vi "Encoder Control Logic.vi"(8 "Prev Phase B (State Bit 1)":bool, 9 "Prev Phase A (State Bit 0)":bool, 10 "Phase B":bool, 11 "Phase A":bool) -> (1 "Count?":bool, 2 "Backward?":bool, 3 "Error Occurred?":bool, 4 "deltaT":i32)   [LabVIEW 2017]
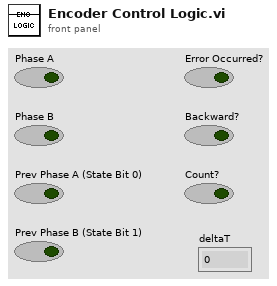
[diagram p1: front panel]
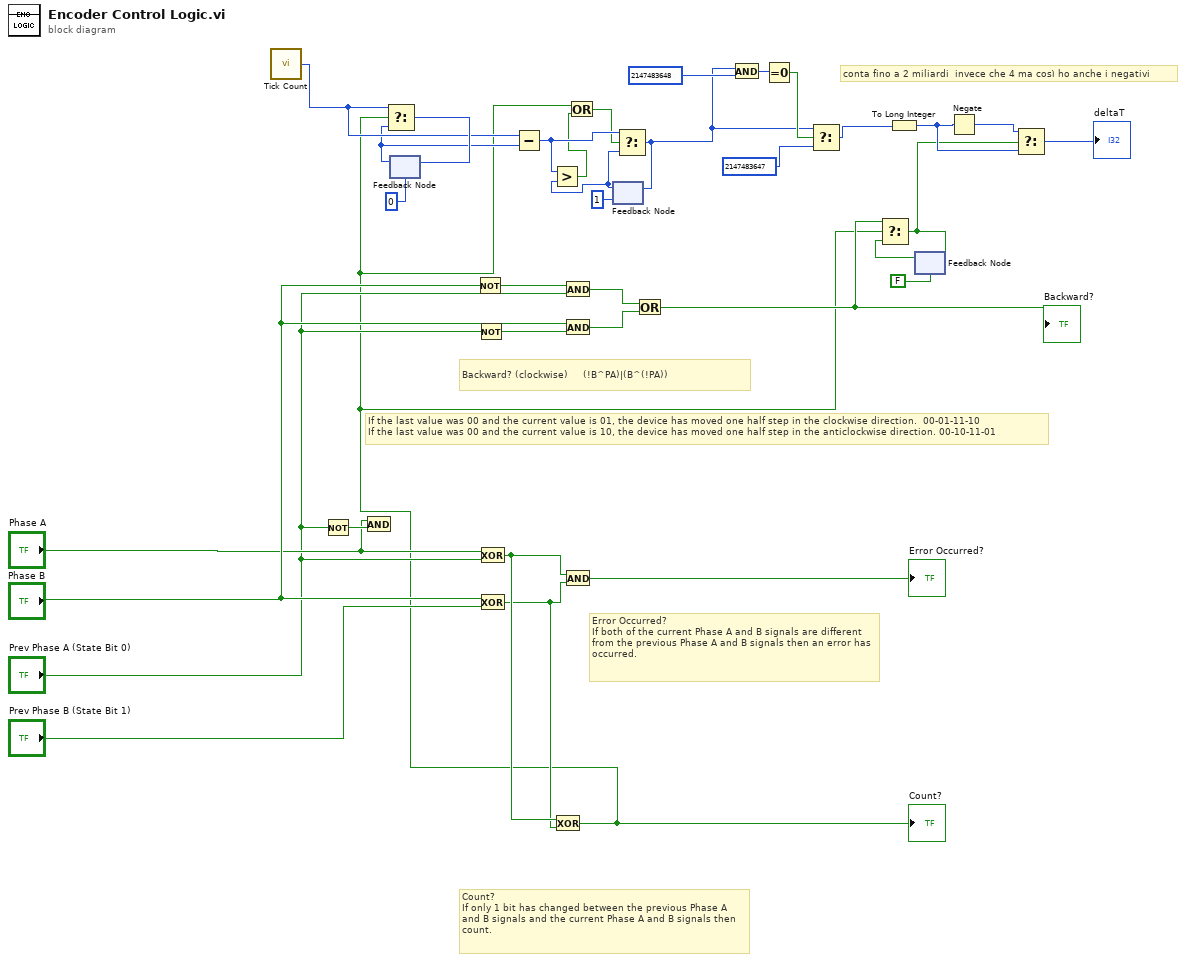
[diagram p0: block diagram]
diagram:
  # "conta fino a 2 miliardi  invece che 4 ma così ho anche i negativi"
  # "If the last value was 00 and the current value is 01, the device has moved one half step in the clockwise direction.  00-01-11-10 \nIf the last value was 00 and the current value is 10, the device has moved one half step in the anticlockwise direction. 00-10-11-01"
  # "Backward? (clockwise)     (!B^PA)|(B^(!PA))"
  # "Count? \nIf only 1 bit has changed between the previous Phase A and B signals and the current Phase A and B signals then count."
  # "Error Occurred?\nIf both of the current Phase A and B signals are different from the previous Phase A and B signals then an error has occurred."
  n1 = call "Tick Count"() -> ("Tick Count(uSec)"=w24:u32)
  n2 = Not(x="Prev Phase A (State Bit 0)") -> (.not. x?=w4:bool)
  n3 = And(x="Phase A", y=w4) -> ()  [unwired: 1 out]
  n4 = feedback #1(u32 0 ("Tick Count(uSec)")) -> (w23:u32)
  n5 = Not(x="Phase B") -> (.not. x?=w35:bool)
  n6 = Not(x="Prev Phase A (State Bit 0)") -> (.not. x?=w34:bool)
  n7 = Exclusive Or(1:"Prev Phase A (State Bit 0)", 2:"Phase A") -> (0:w28:bool)
  n8 = Exclusive Or(1:"Prev Phase B (State Bit 1)", 2:"Phase B") -> (0:w27:bool)
  n9 = Subtract(x=w24, y=w23) -> (x-y=w21:u32)
  n10 = Exclusive Or(1:w27, 2:w28) -> (0:w1:bool)
  "Count?" <- w1
  n11 = Select(t=w24, s=w1, f=w23) -> (s? t:f=w26:u32)
  n12 = feedback-in #1(w26) -> ()
  n13 = And(x=w35, y="Prev Phase A (State Bit 0)") -> (x .and. y?=w32:bool)
  n14 = And(x="Phase B", y=w34) -> (x .and. y?=w33:bool)
  n15 = And(x=w28, y=w27) -> (x .and. y?=→"Error Occurred?":bool)
  n16 = feedback #2(u32 1) -> (w20:u32)
  n17 = Greater?(x=w21, y=w20) -> (0:w18:bool)
  n18 = Or(x=w1, y=w18) -> (x .or. y?=w19:bool)
  n19 = Select(t=w21, s=w19, f=w20) -> (s? t:f=w14:u32)
  n20 = feedback-in #2(w14) -> ()
  n21 = Or(x=w32, y=w33) -> (x .or. y?=w7:bool)
  "Backward?" <- w7
  n22 = And(x=w14, y=u32 2147483648) -> (x .and. y?=w16:u32)
  n23 = Equal To 0?(x=w16) -> (x = 0?=w15:bool)
  n24 = Select(t=w14, s=w15, f=u32 2147483647 ("y")) -> (s? t:f=w11:u32)
  n25 = To Long Integer(number=w11) -> (32bit integer=w10:i32)
  n26 = feedback #3(FALSE) -> (w8:bool)
  n27 = Select(t=w7, s=w1, f=w8) -> (s? t:f=w5:bool)
  n28 = feedback-in #3(w5) -> ()
  n29 = Negate(x=w10) -> (-x=w12:i32)
  n30 = Select(t=w12, s=w5, f=w10) -> (s? t:f=→"deltaT":i32)
